vi "nn symbol.vi"(8 "error in (no error)":errorcluster, 10 "value":i32, 11 "i":i32) -> (0 "error out":errorcluster, 2 "value out":i32, 3 "function return":string)   [LabVIEW 2013, in "lvnano.lvlib"]
doc: "NN_EXPORT const char *nn_symbol (int i, int *value);"
uses:
  lvnano.lvlib
  get last error code.vi
  get error string from code.vi
  <vilib>/Utility/error.llb/Error Cluster From Error Code.vi
  lvnanomsg.dll
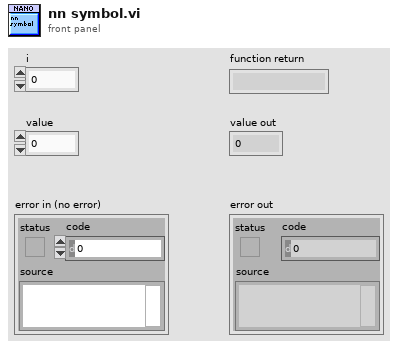
[diagram p1: front panel]
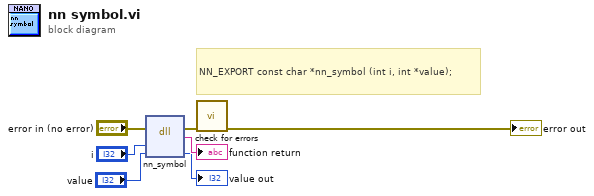
[diagram p0: block diagram]
diagram:
  # "NN_EXPORT const char *nn_symbol (int i, int *value);"
  n1 = dll-call lib="C:/Users/Daniel/Documents/nanomsg/lvnano/lvnanomsg.*" fn="nn_symbol"(error in="error in (no error)", "i"="i", "value"="value") -> (error out=w2:errorcluster, →"function return":string, "value"=→"value out":i32)  [unwired: 3 in, 1 out]
  n2 = call "check for errors.vi"("error in"=w2) -> ("error out"=→"error out":errorcluster)  [unwired: 10 in]
